vi "TestOscilloscope.vi"() -> ()   [LabVIEW 2018]
doc: "This example shows how to configure the oscilloscope to perform an edge-triggered waveform acquisition."
uses:
  Configure Trigger (Edge).vi
  Read (Multiple Waveforms).vi
  Tektronix TDS 200 1000 2000 Series.lvlib
panel:
  out "Numeric":i32
  in  "stop":bool
  in  "Channel (1: Channel 2)":u16(ring) items=["Channel 1", "Channel 2", "Channel 3", "Channel 4", "Math", "Reference A", "Reference B", "Reference C", "Reference D"]
  in  "Channel (0: Channel 1)":u16(ring) items=["Channel 1", "Channel 2", "Channel 3", "Channel 4", "Math", "Reference A", "Reference B", "Reference C", "Reference D"]
  in  "Serial Configuration":T1={"Baud Rate"=9600, "Parity"=0, "Stop Bits"=10, "Flow Control"=0} {"Flow Control" items=["None", "XON/XOFF", "RTS/CTS", "XON/XOFF & RTS/CTS", "DTR/DSR", "XON/XOFF & DTR/DSR"]; "Stop Bits" items=["1.0"=10, "1.5"=15, "2.0"=20]; "Parity" items=["None", "Odd", "Even", "Mark", "Space"]; "Baud Rate" items=["300"=300, "600"=600, "1200"=1200, "2400"=2400, "4800"=4800, "9600"=9600, "19200"=19200]}
  in  "Vertical Coupling (1: DC)":u16(ring)=1 items=["AC", "DC", "Ground"]
  in  "Probe Attenuation (1.0)":dbl=1.0
  in  "Trigger Level (0.0 V)":dbl
  out "Waveform Data":waveform(dbl)[](graph)
  in  "VISA resource name":refnum<visa-resource-name>
  # "(C) 2009-2015 National Instruments.  ALL RIGHTS RESERVED."
  # "To change Vertical Range and Timebase settings, \nplease modify constants on the Block Diagram"
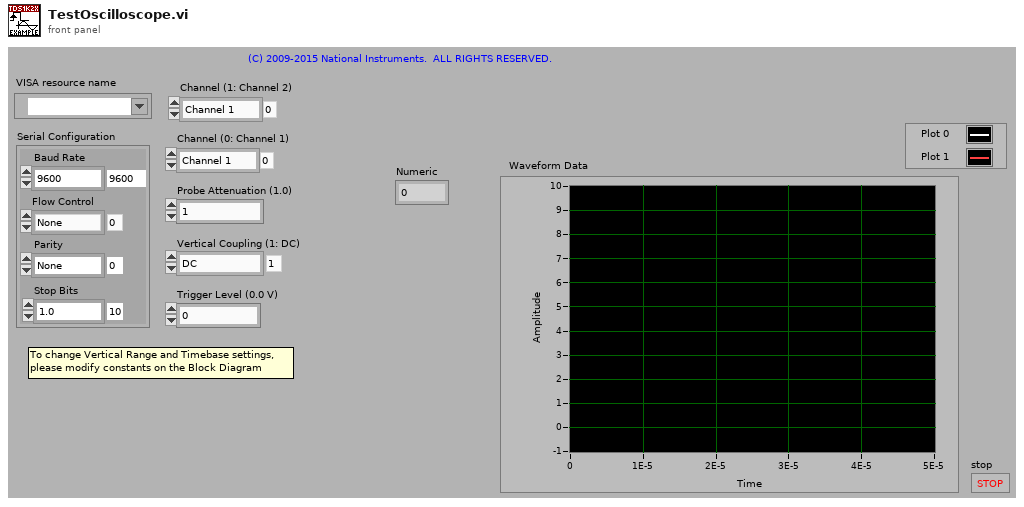
[diagram p1: front panel]
types:
  T1 = cluster{"Baud Rate":u32, "Parity":u16, "Stop Bits":u16, "Flow Control":u16}
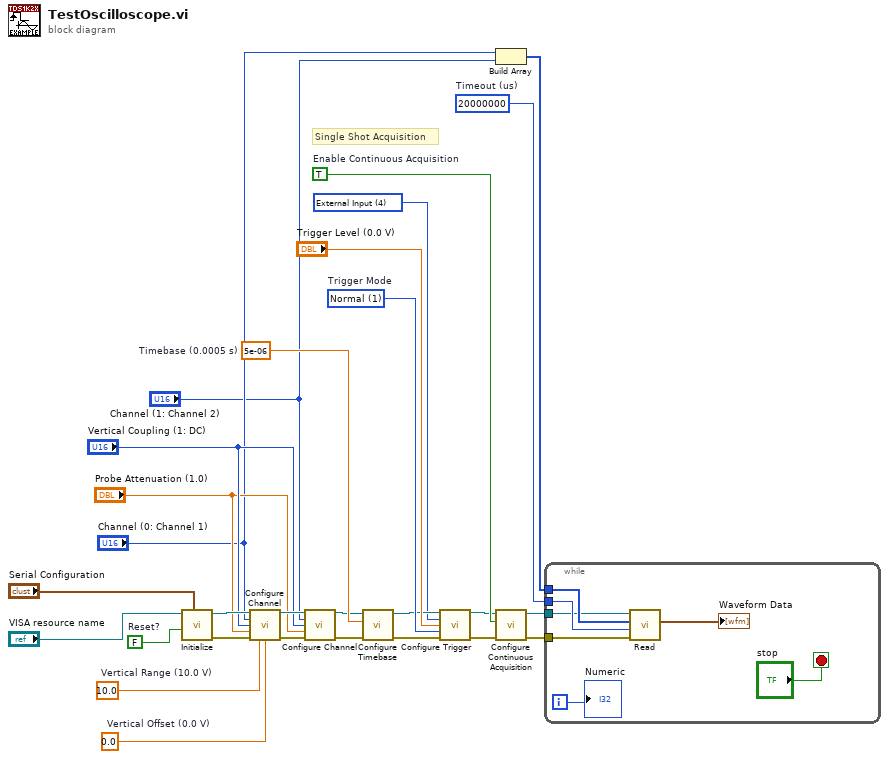
[diagram p0: block diagram]
diagram:
  w9 = 4 items=["Channel 1", "Channel 2", "Channel 3", "Channel 4", "External Input", "Attenuated External Input"] ("Trigger Source (0: Channel 1)")
  w18 = u16 1 items=["Auto", "Normal"]  # Trigger Mode
  w19 = FALSE  # Reset?
  w21 = 0.0  # Vertical Offset (0.0 V)
  w28 = 5e-06  # Timebase (0.0005 s)
  w24 = 10.0  # Vertical Range (10.0 V)
  w3 = u32 20000000  # Timeout (us)
  w23 = TRUE  # Enable Continuous Acquisition
  # "Single Shot Acquisition"
  n1 = call "Initialize.vi"("Serial Configuration"="Serial Configuration", "Reset? (T: Yes)"=w19, "VISA resource name"="VISA resource name") -> ("error out"=w25:errorcluster, "VISA resource name out"=w26:refnum<visa-resource-name>)  [unwired: 2 in, 5 out]
  n2 = call "Configure Channel.vi"("VISA resource name"=w26, "Channel (0: Channel 1)"="Channel (0: Channel 1)", "Vertical Coupling (1: DC)"="Vertical Coupling (1: DC)", "Probe Attenuation (10: 10X)"="Probe Attenuation (1.0)", "error in (no error)"=w25, "Vertical Range (10.0 V/div)"=w24, "Vertical Offset (0.0 divs)"=w21) -> ("VISA resource name out"=w13:refnum<visa-resource-name>, "error out"=w12:errorcluster)  [unwired: 2 in, 5 out]
  n3 = call "Configure Channel.vi"("VISA resource name"=w13, "Channel (0: Channel 1)"="Channel (1: Channel 2)", "Vertical Coupling (1: DC)"="Vertical Coupling (1: DC)", "Probe Attenuation (10: 10X)"="Probe Attenuation (1.0)", "error in (no error)"=w12) -> ("VISA resource name out"=w11:refnum<visa-resource-name>, "error out"=w10:errorcluster)  [unwired: 4 in, 5 out]
  n4 = call "Configure Timebase.vi"("error in (no error)"=w10, "Timebase (0.0005 s)"=w28, "VISA resource name"=w11) -> ("error out"=w16:errorcluster, "VISA resource name out"=w17:refnum<visa-resource-name>)  [unwired: 1 in, 6 out]
  n5 = call-poly "Configure Trigger.vi"("VISA resource name"=w17, "Trigger Source (0: Channel 1)"=w9, "Trigger Level (0.0 V)"="Trigger Level (0.0 V)", "Trigger Mode (0: Auto)"=w18, "error in (no error)"=w16) -> ("VISA resource name out"=w15:refnum<visa-resource-name>, "error out"=w14:errorcluster)  [unwired: 3 in, 6 out]
  n6 = Build Array("Channel (0: Channel 1)", "Channel (1: Channel 2)") -> (w2:u16[])
  n7 = call "Configure Continuous Acquisition.vi"("error in (no error)"=w14, "Enable Continuous Acquisition Mode (True)"=w23, "VISA resource name"=w15) -> ("error out"=w4:errorcluster, "VISA resource name out"=w1:refnum<visa-resource-name>)  [unwired: 7 out]
  n8 = while {
    tunnel: w4 -> [w35]
    tunnel: w3 -> [w34]
    tunnel: w2 -> [w33]
    tunnel: w1 -> [w32]
    i -> [w29]
    stop <- "stop" stop-if-true
    n9 = call-poly "Read.vi"("error in (no error)"=w35, "Timeout (10000 ms)"=w34, "Channels"=w33, "VISA resource name"=w32) -> ("Waveform Data"=→"Waveform Data":waveform(dbl)[])  [unwired: 7 out]
    "Numeric" <- w29
  }
